vi "Set Reference Sinusoidal Fit.vi"(8 "error in (no error)":errorcluster, 10 "Sinusoidal Fit.lvclass":refnum<class "Sinusoidal Fit.lvclass">, 11 "Halfwave Sinusoidal Fit in":refnum<class "Halfwave Sinusoidal Fit.lvclass">) -> (0 "error out":errorcluster, 3 "Halfwave Sinusoidal Fit out":refnum<class "Halfwave Sinusoidal Fit.lvclass">)   [LabVIEW 2016, in "Halfwave Sinusoidal Fit.lvclass"]
uses:
  Halfwave Sinusoidal Fit.lvclass
  Sinusoidal Fit.lvclass
  Halfwave Sinusoidal Fit.lvclass/Halfwave Sinusoidal Fit.ctl
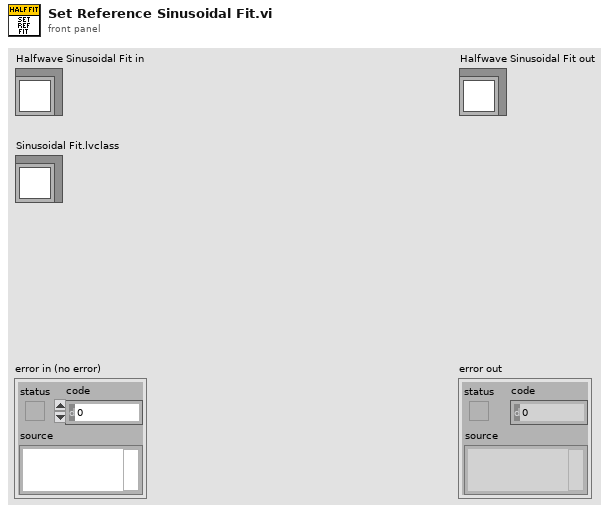
[diagram p1: front panel]
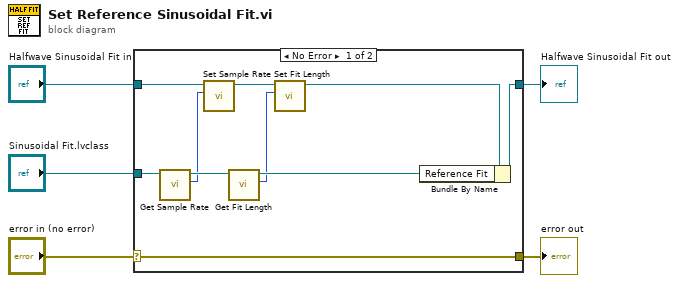
[diagram p0: block diagram]
diagram:
  n1 = case shown="No Error" "error in (no error)" {
    selector: "error in (no error)" -> [w15 w16]
    tunnel: [w15 w16] -> w4
    tunnel: [w14 w17] -> w2
    tunnel: "Halfwave Sinusoidal Fit in" -> [w9 w17]
    tunnel: "Sinusoidal Fit.lvclass" -> [w13 _]
    frame No Error {
      n2 = call-dynamic "Get Sample Rate.vi"("Abstract Fit in"=w13) -> ("Sample Rate"=w7:i32, "Abstract Fit out"=w12:refnum<class "Sinusoidal Fit.lvclass">)  [unwired: 8 in, 1 out]
      n3 = call-dynamic "Set Sample Rate.vi"("Sample Rate"=w7, "Abstract Fit in"=w9) -> ("Abstract Fit out"=w10:refnum<class "Halfwave Sinusoidal Fit.lvclass">)  [unwired: 8 in, 1 out]
      n4 = call-dynamic "Get Fit Length.vi"("Abstract Fit in"=w12) -> ("Length"=w6:i32, "Abstract Fit out"=w11:refnum<class "Sinusoidal Fit.lvclass">)  [unwired: 8 in, 1 out]
      n5 = call-dynamic "Set Fit Length.vi"("Length"=w6, "Abstract Fit in"=w10) -> ("Abstract Fit out"=w8:refnum<class "Halfwave Sinusoidal Fit.lvclass">)  [unwired: 8 in, 1 out]
      n6 = Bundle By Name(cluster=w8, "Reference Fit"=w11) -> (w14:refnum<class "Halfwave Sinusoidal Fit.lvclass">)
    }
    frame Error {
    }
  }
  "error out" <- w4
  "Halfwave Sinusoidal Fit out" <- w2
